vi "SetHint.vi"(8 "No Error":errorcluster, 10 "Value":string, 11 "Hint Name":T1) -> (0 "error out":errorcluster)   [LabVIEW 2024, in "SDL3.lvlib" / "Hints.lvlib"]
doc: "<B>Summary</B>\nSet a hint with normal priority.\n\n<B>Remarks</B>\nHints will not be set if there is an existing override hint or environment variable that takes precedence. You can use <B>SDL_SetHintWithPriority()</B> to set the hint with override priority instead."
uses:
  Hints.lvlib
  Lib/Win32/SDL3.dll
  HintName--combobox.ctl
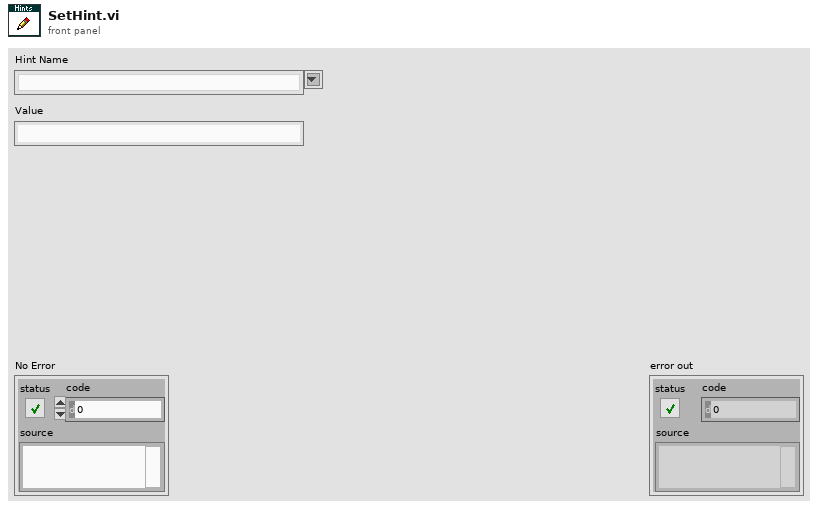
[diagram p1: front panel]
types:
  T1 = typedef "SDL3.lvlib/Hints.lvlib/HintName--combobox.ctl" = string
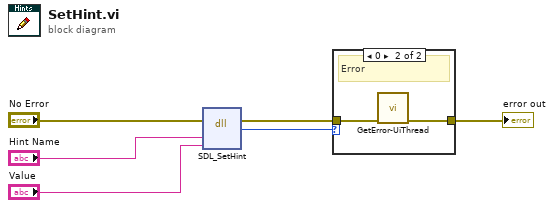
[diagram p0: block diagram]
diagram:
  n1 = dll-call lib="C:/Users/Thomas/Documents/Projects/LV-SDL3/Lib/Win32/SDL3.dll" fn="SDL_SetHint"(error in="No Error", "name"="Hint Name", "value"="Value") -> (error out=w3:errorcluster, "return type"=w1:i32)  [unwired: 4 in, 1 out]
  n2 = case shown="0" w1 {
    tunnel: w3 -> [w7 w9]
    tunnel: [w7 w8] -> w2
    frame Default {
      # "Ok"
    }
    frame 0 {
      # "Error"
      n3 = call "GetError-UiThread.vi"("No Error"=w9) -> ("error out"=w8:errorcluster)  [unwired: 10 in]
    }
  }
  "error out" <- w2
